vi "Test_sqlite3Open_worksNoError.vi"(8 "error in (no error)":errorcluster, 11 "TestCase in":refnum<class "Test sqlite3.lvclass">) -> (0 "error out":errorcluster, 3 "TestCase out":refnum<class "Test sqlite3.lvclass">)   [LabVIEW 2020, in "Test sqlite3.lvclass"]
uses:
  Test sqlite3.lvclass
  externals/sqlite3/Source/sqlite3.lvclass/sqlite3.ctl
  <vilib>/Utility/error.llb/Error Cluster From Error Code.vi
  externals/sqlite3/Source/sqlite3.lvclass
  <vilib>/addons/_JKI Toolkits/VI Tester/TestCase.llb/TestCase.lvclass
  C:/Program Files/National Instruments/LabVIEW 2020/vi.lib/addons/_JKI Toolkits/VI Tester/TestCase.llb/TestCase.lvclass
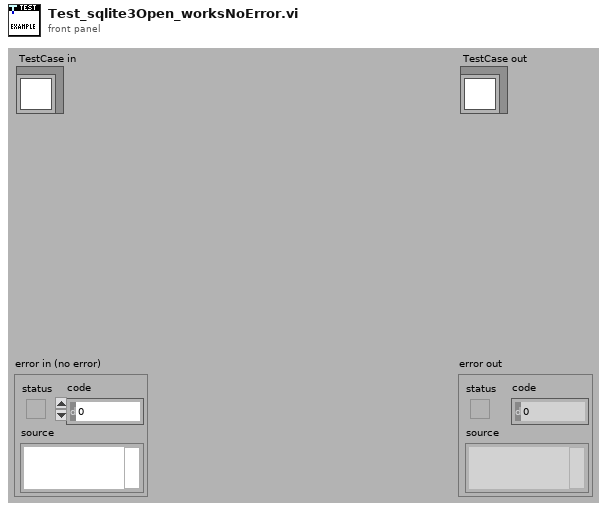
[diagram p1: front panel]
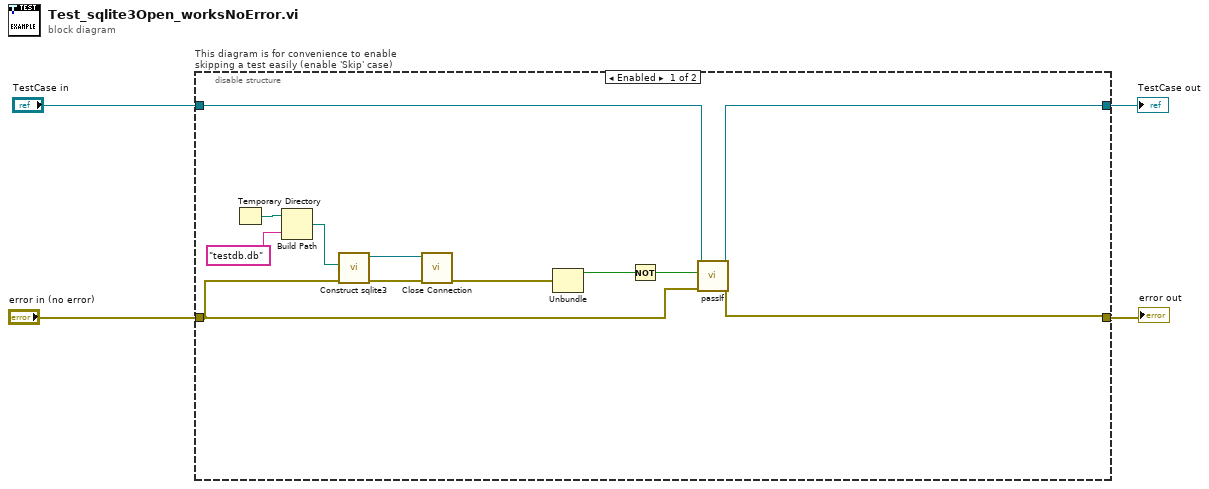
[diagram p0: block diagram]
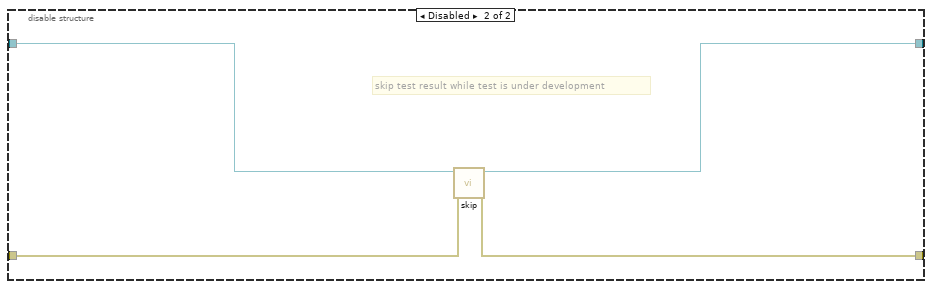
[diagram p2: hidden frame]
diagram:
  n1 = disable-structure "This diagram is for convenience to enable skipping a test easily (enable 'Skip' case)" shown="Enabled" {
    disable-tunnel: "TestCase in" -> [w16 w20]
    disable-tunnel: [w15 w18] -> w1
    disable-tunnel: [w14 w19] -> w3
    disable-tunnel: "error in (no error)" -> [w13 w17]
    frame Enabled {
      n2 = Temporary Directory() -> (w9:path)
      n3 = Build Path(base path=w9, name or relative path="testdb.db") -> (appended path=w7:path)
      n4 = call "Construct sqlite3.vi"("error in (no error)"=w13, "DatabaseFilePath"=w7) -> ("error out"=w6:errorcluster, "sqlite3 out"=w5:refnum<class "sqlite3.lvclass">)  [unwired: 8 in]
      n5 = call-dynamic "Close Connection.vi"("error in (no error)"=w6, "sqlite in"=w5) -> ("error out"=w10:errorcluster)  [unwired: 8 in, 1 out]
      n6 = Unbundle(w10) -> ("status"=w12:bool)  [unwired: 2 out]
      n7 = Not(x=w12) -> (.not. x?=w11:bool)
      n8 = call-dynamic "passIf.vi"("error in (no error)"=w13, "pass"=w11, "TestCase in"=w16) -> ("error out"=w14:errorcluster, "TestCase out"=w15:refnum<class "Test sqlite3.lvclass">)  [unwired: 7 in]
    }
    frame Disabled {
      # "skip test result while test is under development"
      n9 = call <vilib>:"skip.vi"("error in (no error)"=w17, "TestCase in"=w20) -> ("error out"=w19:errorcluster, "TestCase out"=w18:refnum<class "Test sqlite3.lvclass">)  [unwired: 8 in]
    }
  }
  "error out" <- w3
  "TestCase out" <- w1
